vi "Servo Camera.vi"() -> ()   [LabVIEW 2013]
doc: "<B>Servo Camera Example</B> will track a colored object by moving a gimbal mounted camera to keep the object centered in the image. It assumes the camera is mounted upright, and that the DS is connected. It is written to control two servos, but will work fine with one. To tune the colors, you may find it easiest to set the Operation control to Camera Display. This way the servos will not update and you can experiment with the colors to get a good mask.\nOnce the color thresholds are set appropriately for the object you are tracking, switch Operation to GimbalTrack."
uses:
  <vilib>/addons/control/pid/NI_PID_pid.lvlib
  <vilib>/addons/control/pid/pid.llb/PID Control Input Filter (DBL).vi
  <vilib>/Rock Robotics/WPI/Camera/WPI_CameraFrameRate.ctl
  <vilib>/Rock Robotics/WPI/Camera/WPI_CameraImageSize.ctl
  Control States.ctl
  <vilib>/Rock Robotics/SystemInterfaces/DIO/FPGA_DIOPWMChannel.ctl
  2014 Target Detection/TargetType.ctl
panel:
  out "x = y?":cluster{bool, bool, bool, bool}
  in  "Color Components":T1={"Hue"={112.66304016113281, 144.6630401611328}, "Sat"={138.0, 255.0}, "Val"={139.0, 198.0}} {"Val" scale=0.0..255.0; "Sat" scale=0.0..255.0; "Hue" scale=0.0..255.0 scale format="%#_3g"}
  in  "Std Devs":cluster{"Hue":dbl, "Sat":dbl, "Val":dbl}={"Hue"=4.0, "Sat"=6.0, "Val"=4.0}
  out "Target Info":T3(array[cluster])
  in  "Score Cutoff":dbl(slide)=54.248366013071895 scale=0.0..100.0
  in  "Area Size Limit %":dbl=0.06 format="%#_13g"
  out "Image":T4(plugin-control)
  in  "stop":bool
  in  "Operation":enum32{"Camera Display", "Gimbal Track"}(radio)
  out "Servo Tracking State":T6
  in  "Servo Positions":cluster{"X":dbl, "Y":dbl}={"X"=85.52840986947938, "Y"=85.0} {"Y" scale=0.0..170.0; "X" scale=0.0..170.0}
  in  "Y Channel":T7=enum."PWM 5"
  in  "Loop Sleep":u32=20
  in  "Loop Sleep":u32=80
  in  "X Channel":T7=enum."PWM 4"
  in  "Image Decimation":cluster{"X":dbl, "Y":dbl}={"X"=5.0, "Y"=4.0}
  in  "Color Ranges":T8={"Hue"={"Min"=55, "Max"=93}, "Sat"={"Min"=41, "Max"=255}, "Luma"={"Min"=64, "Max"=255}}
  in  "Smooth":bool=TRUE
  out "Mask after threshold":T4(plugin-control)
  in  "Display Mask":bool=TRUE
  out "Camera Image":T4(plugin-control)
  # "This example will track a colored object by moving a gimbal mounted camera to keep the object centered in the image. It assumes the camera is mounted upright, and that the DS is connected. It is written to control two servos, but will work fine with one. To tune the colors, you may find it easiest to set the Operation control to Camera Display. This way the servos will not update and you can experiment with the colors to get a good mask.\nOnce the color thresholds are set appropriately for the object you are tracking, switch Operation to GimbalTrack."
  # "Servo Settings"
  # "Camera Settings"
  # "Hues are ~ 70, 150, and 250\nfor Green, Blue, and Red."
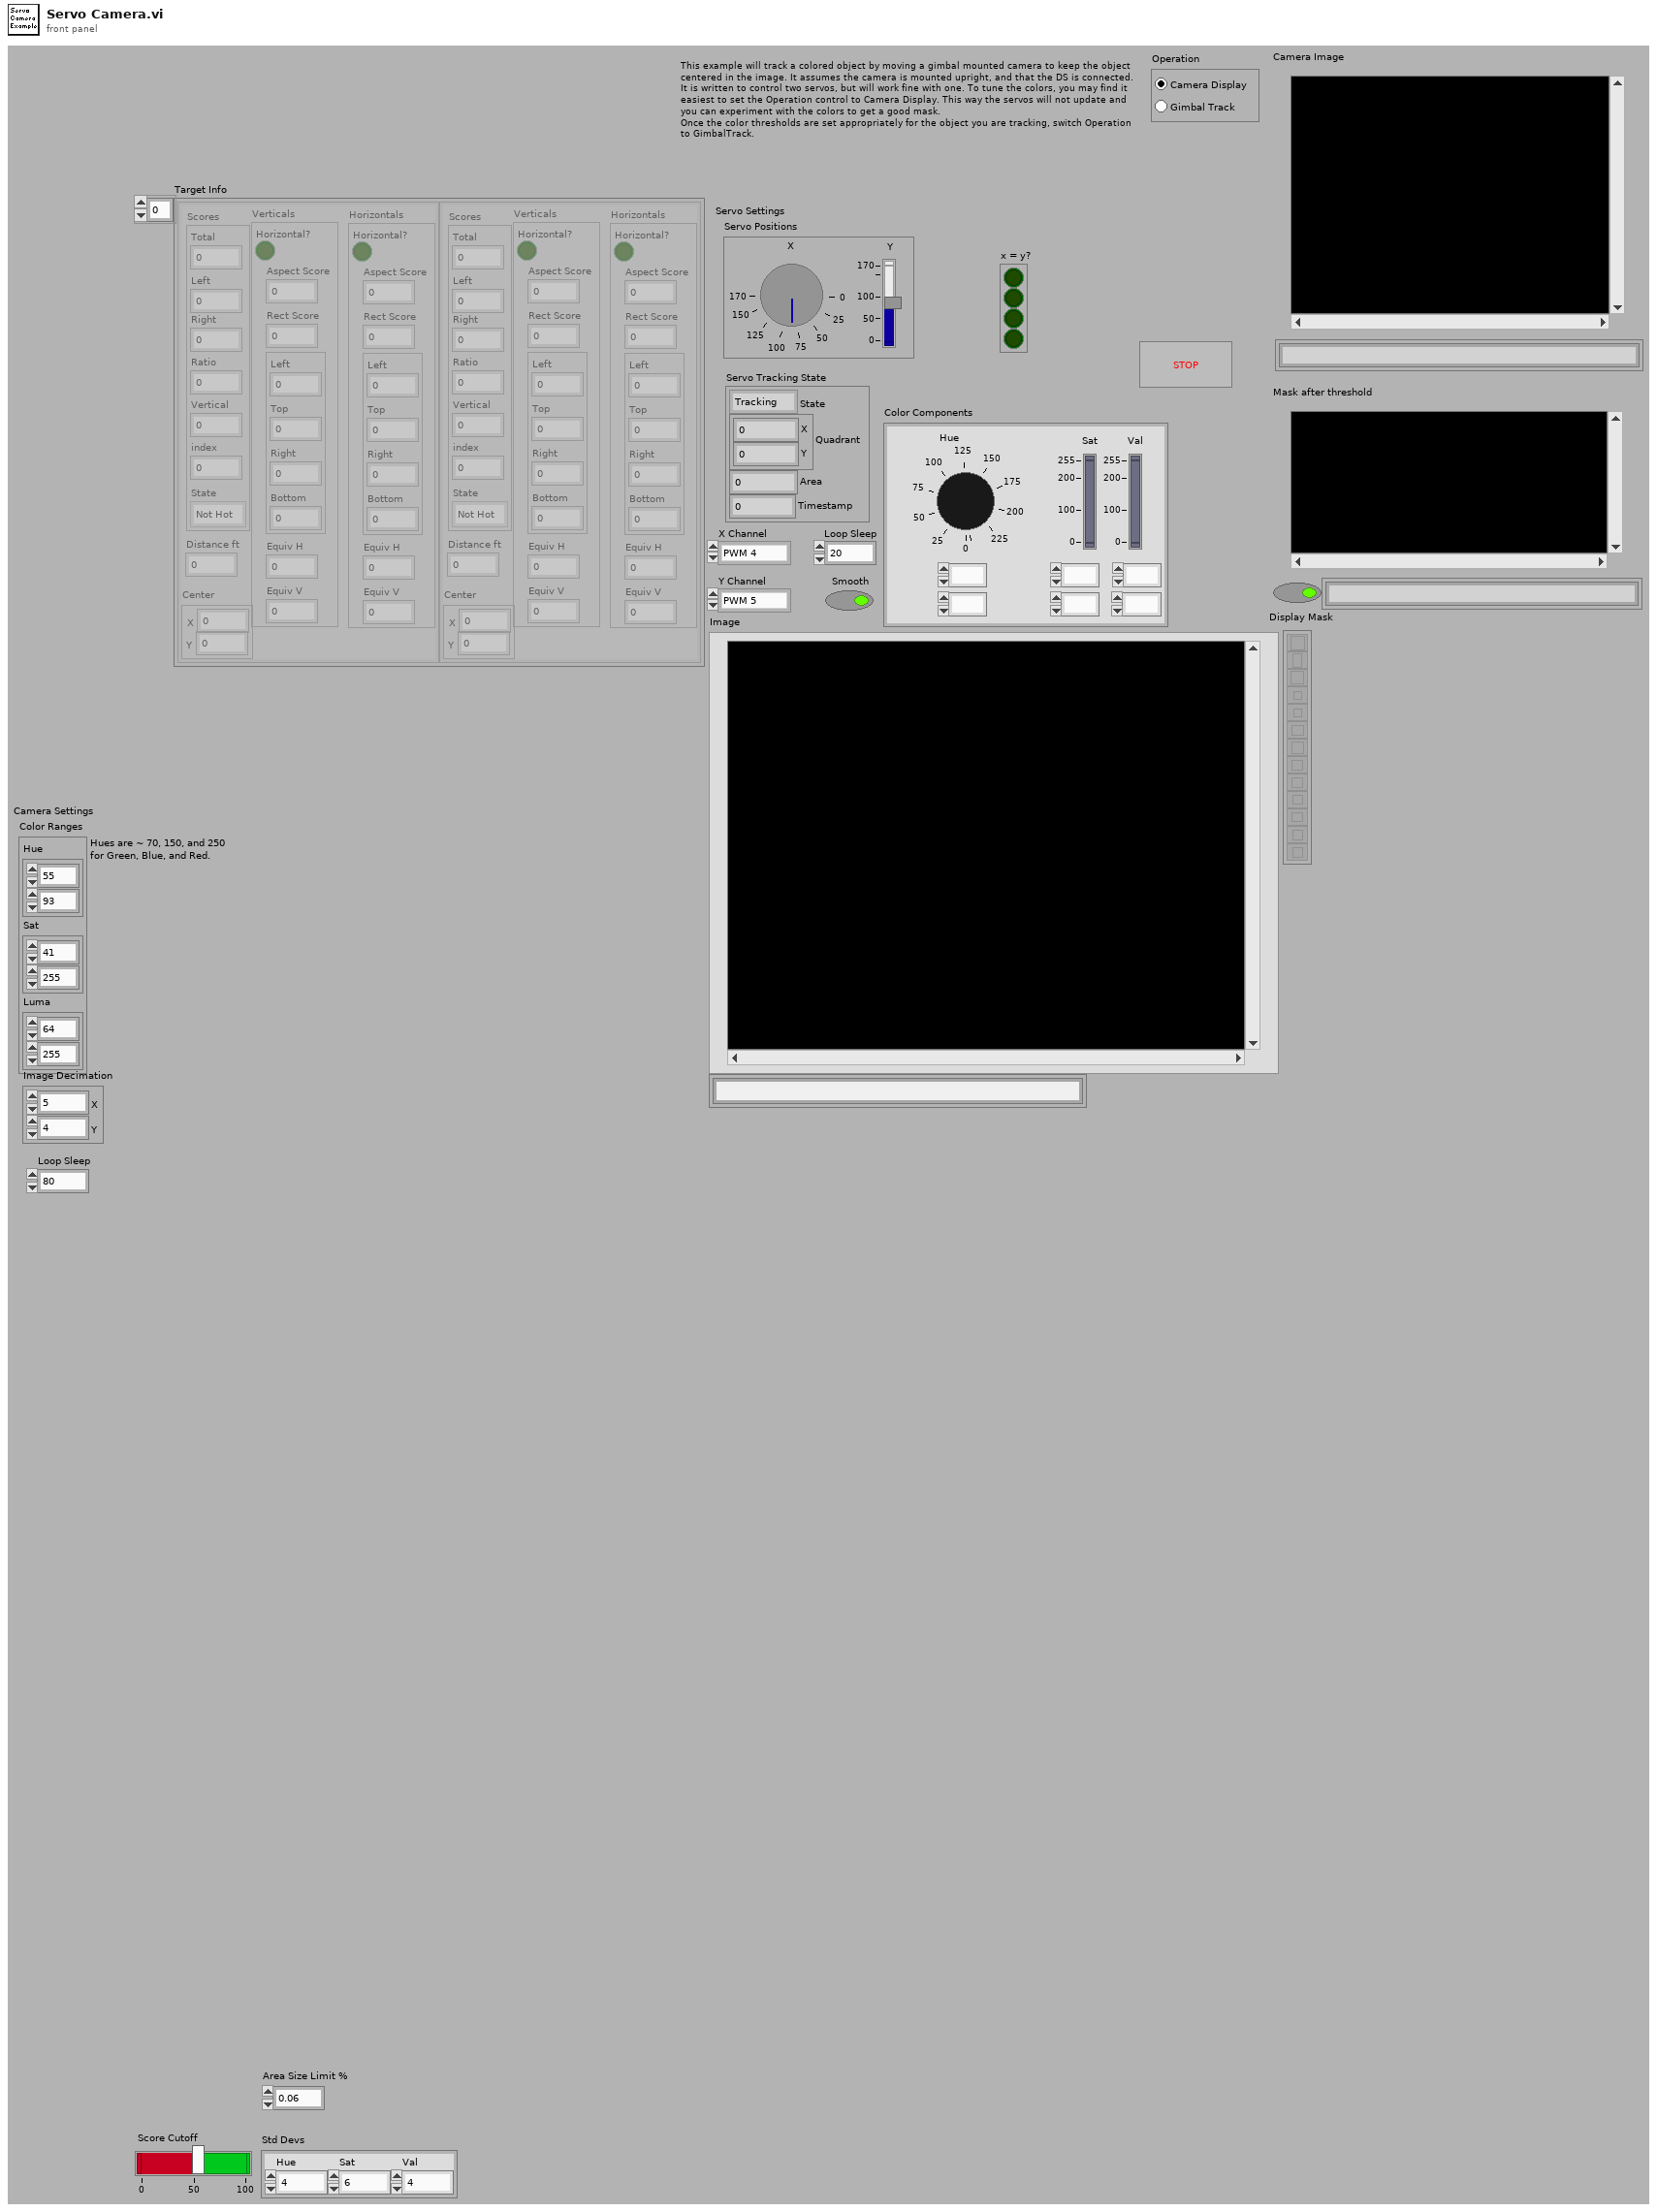
[diagram p1: front panel]
types:
  T1 = cluster{"Hue":cluster{dbl, dbl}, "Sat":cluster{dbl, dbl}, "Val":cluster{dbl, dbl}}
  T2 = typedef "TargetType.ctl" = enum16{"Not Hot", "Hot"}
  T3 = cluster{"Scores":cluster{"Total":dbl, "Left":dbl, "Right":dbl, "Ratio":dbl, "Vertical":dbl, "index":i32, "State":T2}, "Verticals":cluster{"Horizontal?":bool, "Aspect Score":dbl, "Rect Score":dbl, cluster{"Left":dbl, "Top":dbl, "Right":dbl, "Bottom":dbl}, "Equiv H":dbl, "Equiv V":dbl}, "Horizontals":cluster{"Horizontal?":bool, "Aspect Score":dbl, "Rect Score":dbl, cluster{"Left":dbl, "Top":dbl, "Right":dbl, "Bottom":dbl}, "Equiv H":dbl, "Equiv V":dbl}, "Distance ft":dbl, "Center":cluster{"X":dbl, "Y":dbl}}[]
  T4 = typedef "IMAQ Image.ctl" = refnum<image>
  T5 = typedef "Control States.ctl" = enum16{"Tracking", "Lost Small", "Lost-Patience", "Search-Begin", "Searching", "Lost - Edge"}
  T6 = cluster{"State":T5, "Quadrant":cluster{"X":i32, "Y":i32}, "Area":i32, "Timestamp":u32}
  T7 = typedef "FPGA_DIOPWMChannel.ctl" = enum8{"PWM 1", "PWM 2", "PWM 3", "PWM 4", "PWM 5", "PWM 6", "PWM 7", "PWM 8", "PWM 9", "PWM 10", "Invalid"}
  T8 = cluster{"Hue":cluster{"Min":i32, "Max":i32}, "Sat":cluster{"Min":i32, "Max":i32}, "Luma":cluster{"Min":i32, "Max":i32}}
  T9 = typedef "WPI_CameraImageSize.ctl" = enum16{"640x480", "320x240", "160x120"}
  T10 = typedef "WPI_CameraFrameRate.ctl" = u32
  T11 = typedef "WPI_CameraDevRef.ctl" = cluster{"Camera Address":string, "CameraStatus":errorcluster, "Acquire Image Notifier":refnum<notifier>}
  T12 = typedef "WPI_ServoDeviceRef.ctl" = cluster{"DeviceStatus":errorcluster, "Digital Module":T13, "PWM Channel":T7, "DeadBand":T14}
  T13 = typedef "FPGA_TypedefDigitalModule.ctl" = enum16{"Digital Module 1", "Digital Module 2"}
  T14 = typedef "WPI_PWMDeadband.ctl" = cluster{"Name":string, "maxPositivePwm":i32, "minPositivePwm":i32, "centerPwm":i32, "maxNegativePwm":i32, "minNegativePwm":i32, "angularRange":u16}
  T15 = cluster{"Left":i32, "Top":i32, "Right":i32, "Bottom":i32}
  T16 = cluster{"Horizontal":bool, "Aspect Score":dbl, "Rect Score":dbl, cluster{"Left":dbl, "Top":dbl, "Right":dbl, "Bottom":dbl}, "Equiv H":dbl, "Equiv V":dbl}[]
  T17 = cluster{cluster{dbl, dbl}, cluster{dbl, dbl}, cluster{dbl, dbl}}
  T18 = cluster{"Scores":cluster{"Total":dbl, "Left":dbl, "Right":dbl, "Ratio":dbl, "Vertical":dbl, "index":i32, "State":T2}, "Verticals":cluster{"Horizontal?":bool, "Aspect Score":dbl, "Rect Score":dbl, cluster{"Left":dbl, "Top":dbl, "Right":dbl, "Bottom":dbl}, "Equiv H":dbl, "Equiv V":dbl}, "Horizontals":cluster{"Horizontal?":bool, "Aspect Score":dbl, "Rect Score":dbl, cluster{"Left":dbl, "Top":dbl, "Right":dbl, "Bottom":dbl}, "Equiv H":dbl, "Equiv V":dbl}, "Validated":bool}[]
  T19 = cluster{"Distance (ft)":dbl, "Target Center (-1 to 1)":cluster{"X":dbl, "Y":dbl}, "Left":bool, "State":T2}[]
  T20 = cluster{"Scores":cluster{"Total":dbl, "Left":dbl, "Right":dbl, "Ratio":dbl, "Vertical":dbl, "index":i32, "State":T2}, "Verticals":cluster{"Horizontal?":bool, "Aspect Score":dbl, "Rect Score":dbl, cluster{"Left":dbl, "Top":dbl, "Right":dbl, "Bottom":dbl}, "Equiv H":dbl, "Equiv V":dbl}, "Horizontals":cluster{"Horizontal?":bool, "Aspect Score":dbl, "Rect Score":dbl, cluster{"Left":dbl, "Top":dbl, "Right":dbl, "Bottom":dbl}, "Equiv H":dbl, "Equiv V":dbl}, "Distance (ft)":dbl, "Target Center (-1 to 1)":cluster{"X":dbl, "Y":dbl}}[]
  T21 = cluster{"Scores":cluster{"Total":dbl, "Left":dbl, "Right":dbl, "Ratio":dbl, "Vertical":dbl, "index":i32, "State":T2}, "Verticals":cluster{"Horizontal?":bool, "Aspect Score":dbl, "Rect Score":dbl, cluster{"Left":dbl, "Top":dbl, "Right":dbl, "Bottom":dbl}, "Equiv H":dbl, "Equiv V":dbl}, "Horizontals":cluster{"Horizontal?":bool, "Aspect Score":dbl, "Rect Score":dbl, cluster{"Left":dbl, "Top":dbl, "Right":dbl, "Bottom":dbl}, "Equiv H":dbl, "Equiv V":dbl}, "Distance (ft)":dbl, "Target Center (-1 to 1)":cluster{"X":dbl, "Y":dbl}}
  T22 = cluster{"Horizontal?":bool, "Aspect Score":dbl, "Rect Score":dbl, cluster{"Left":dbl, "Top":dbl, "Right":dbl, "Bottom":dbl}, "Equiv H":dbl, "Equiv V":dbl}
  T23 = cluster{"Distance (ft)":dbl, "Target Center (-1 to 1)":cluster{"X":dbl, "Y":dbl}, "Left":bool, "State":T2}
  T24 = cluster{"Left":dbl, "Top":dbl, "Right":dbl, "Bottom":dbl}
  T25 = cluster{"State":T5, "Quadrant":cluster{"X":i32, "Y":i32}, "Area":i32, "millisecond timer value":u32}
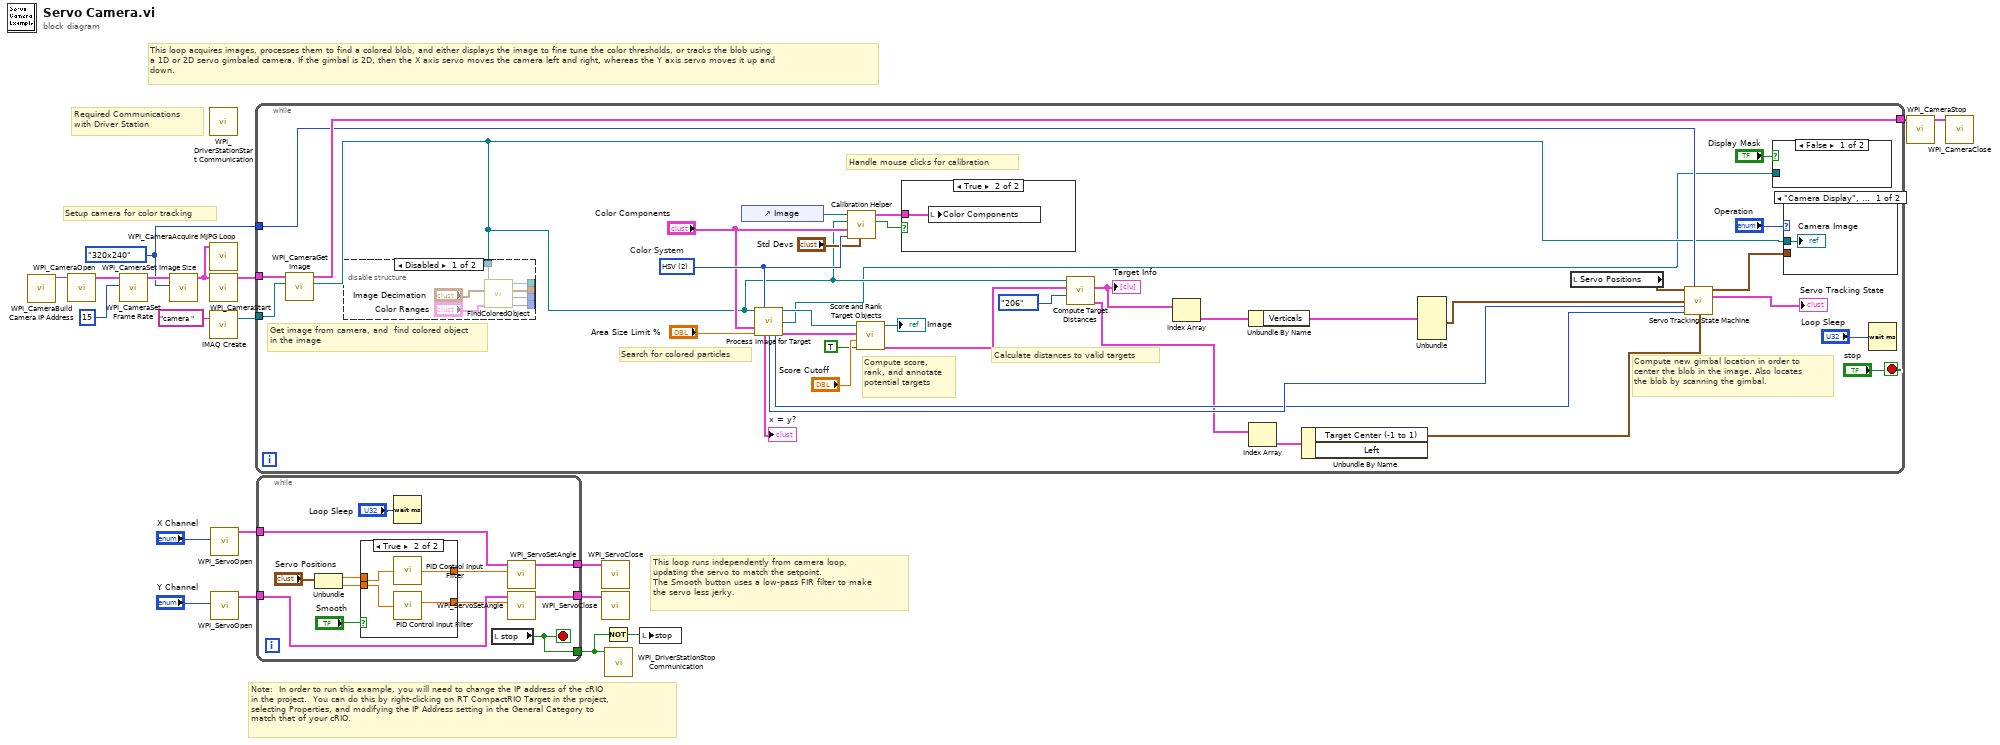
[diagram p0: block diagram]
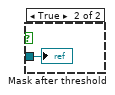
[diagram p4: hidden frame]
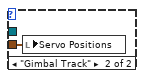
[diagram p5: hidden frame]
diagram:
  w7 = WPI_CameraImageSize."320x240" ("Image Size")
  # "Note:  In order to run this example, you will need to change the IP address of the cRIO\nin the project.  You can do this by right-clicking on RT CompactRIO Target in the project,\nselecting Properties, and modifying the IP Address setting in the General Category to \nmatch that of your cRIO."
  # "This loop acquires images, processes them to find a colored blob, and either displays the image to fine tune the color thresholds, or tracks the blob using\na 1D or 2D servo gimbaled camera. If the gimbal is 2D, then the X axis servo moves the camera left and right, whereas the Y axis servo moves it up and\ndown."
  # "This loop runs independently from camera loop,\nupdating the servo to match the setpoint.\nThe Smooth button uses a low-pass FIR filter to make\nthe servo less jerky."
  # "Setup camera for color tracking"
  # "Required Communications\nwith Driver Station"
  n1 = call <vilib>:"WPI_CameraBuild Camera IP Address.vi"() -> ("Camera Address"=w4:string)  [unwired: 11 in]
  n2 = call <vilib>:"WPI_CameraOpen.vi"("Camera Address"=w4) -> ("CameraDevRef"=w8:T11)  [unwired: 1 in, 9 out]
  n3 = call <vilib>:"WPI_CameraSet Frame Rate.vi"("Frame Rate (fps)"=T10 15, "CameraDevRef"=w8) -> ("CameraDevRef Out"=w9:T11)  [unwired: 1 in, 8 out]
  n4 = call <vilib>:"WPI_CameraSet Image Size.vi"("Image Size"=w7, "CameraDevRef"=w9) -> ("CameraDevRef Out"=w3:T11)  [unwired: 1 in, 8 out]
  n5 = call <vilib>:"WPI_DriverStationStart Communication.vi"() -> ()  [unwired: 1 in, 11 out]
  n6 = call <vilib>:"WPI_CameraAcquire MJPG Loop.vi"("CameraDevRef"=w3) -> ()  [unwired: 11 in]
  n7 = call <vilib>:"WPI_CameraStart.vi"("CameraDevRef"=w3) -> ("CameraDevRef Out"=w12:T11)  [unwired: 1 in, 9 out]
  n8 = call "IMAQ Create"("Image Name"="camera ") -> ("New Image"=w13:T4)  [unwired: 3 in, 2 out]
  n9 = call <vilib>:"WPI_ServoOpen.vi"("PWM Channel"="X Channel") -> ("ServoDeviceRef"=w17:T12)  [unwired: 3 in, 7 out]
  n10 = call <vilib>:"WPI_ServoOpen.vi"("PWM Channel"="Y Channel") -> ("ServoDeviceRef"=w16:T12)  [unwired: 3 in, 7 out]
  n11 = while {
    tunnel: w12 -> [w52]
    tunnel: [w51] -> w11
    tunnel: w13 -> [w55]
    tunnel: w7 -> [w46]
    stop <- "stop" stop-if-true
    w37 = u16 2 items=["RGB", "HSL", "HSV", "HSI"]  # Color System
    # "Calculate distances to valid targets"
    # "Search for colored particles"
    # "Handle mouse clicks for calibration"
    # "Compute score,\nrank, and annotate\npotential targets"
    # "Compute new gimbal location in order to\ncenter the blob in the image. Also locates\nthe blob by scanning the gimbal."
    # "Get image from camera, and  find colored object in the image"
    n12 = call <vilib>:"WPI_CameraGet Image.vi"("Image"=w55, "CameraDevRef"=w52) -> ("Image Out"=w31:T4, "CameraDevRef Out"=w51:T11)  [unwired: 1 in, 7 out]
    n13 = disable-structure shown="Disabled" {
      disable-tunnel: [w64 _] -> _
      disable-tunnel: [w63 _] -> _
      disable-tunnel: [w62 _] -> _
      disable-tunnel: [w59 _] -> _
      disable-tunnel: w31 -> [w58 _]
      frame Disabled {
        n14 = call "FindColoredObject.vi"("Color Range"="Color Ranges", "Decimate by"="Image Decimation", "Color Image In"=w58) -> ("Area"=w62:i32, "Particles"=w63:i32, "Rectangle"=w64:T15, "Mask Image"=w59:T4)  [unwired: 3 out]
      }
      frame Enabled {
      }
    }
    n15 = control-ref of="Image"() -> (w38:refnum<vi>)
    n16 = call "Process Image for Target.vi"("Src Image"=w31, "Color Mode"=w37, "Color Components"="Color Components", "Area Cutoff %"="Area Size Limit %") -> ("Src Image Out"=w44:T4, "Threshold"=w30:T4, "x = y?"=→"x = y?":cluster{bool, bool, bool, bool}, "Particles gimbal"=w25:i32, "area"=w24:i32, "Particles"=w41:T16)  [unwired: 6 in]
    n17 = call "Calibration Helper.vi"("Std Devs"="Std Devs", "Color Mode"=w37, "Color Components"="Color Components", "Image"=w31, "Image Ctl Refnum"=w38) -> ("Changed"=w33:bool, "output color"=w35:T17)  [unwired: 5 in]
    n18 = call "Score and Rank Target Objects.vi"("Annotate"=TRUE, "Score Limit"="Score Cutoff", "Particles"=w41, "Image in"=w44) -> ("Target Info"=w40:T18, "Annotated Image"=→"Image":T4)  [unwired: 6 in]
    n19 = case shown="True" w33 {
      tunnel: w35 -> [_ w57]
      frame False {
      }
      frame True {
        n20 = local write "Color Components"(w57) -> ()
      }
    }
    n21 = call "Compute Target Distances.vi"("Camera Type"=enum16{"206", "1011", "1013"}."206", "Target Info"=w40, "Image in"=w31) -> ("Distances"=w22:T19, "Target Info"=w29:T20)  [unwired: 6 in, 1 out]
    "Target Info" <- w29
    n22 = Index Array(array=w29) -> (element=w28:T21)  [unwired: 1 in]
    n23 = Unbundle By Name(w28) -> ("Verticals"=w27:T22)
    n24 = Index Array(array=w22) -> (element=w21:T23)  [unwired: 1 in]
    n25 = Unbundle By Name(w21) -> ("Target Center (-1 to 1)"=w20:cluster{"X":dbl, "Y":dbl})  [unwired: 1 out]
    n26 = Unbundle(w27) -> (w26:T24)  [unwired: 5 out]
    n27 = local read "Servo Positions"() -> (w50:cluster{"X":dbl, "Y":dbl})
    n28 = call "Servo Tracking State Machine.vi"("Servo Positions In"=w50, "Image Size"=w46, "Rectangle"=w26, "Particles"=w25, "Area"=w24, "Center"=w20) -> ("Servo Positions"=w54:cluster{"X":dbl, "Y":dbl}, "Tracking State Info"=→"Servo Tracking State":T25)  [unwired: 1 in, 7 out]
    n29 = case shown="False" "Display Mask" {
      tunnel: w30 -> [_ w65]
      frame False {
      }
      frame True {
        "Mask after threshold" <- w65
      }
    }
    n30 = case shown="\"Camera Display\", Default" "Operation" {
      tunnel: w54 -> [_ w67]
      tunnel: w31 -> [w66 _]
      frame "Camera Display", Default {
        "Camera Image" <- w66
      }
      frame "Gimbal Track" {
        n31 = local write "Servo Positions"(w67) -> ()
      }
    }
    n32 = Wait (ms)(milliseconds to wait="Loop Sleep") -> ()  [unwired: 1 out]
  }
  n33 = while {
    tunnel: w17 -> [w77]
    tunnel: [w79] -> w6
    tunnel: w16 -> [w76]
    tunnel: [w75] -> w5
    tunnel: [w68] -> w2
    stop <- w68 stop-if-true
    n34 = Unbundle("Servo Positions") -> ("X"=w73:dbl, "Y"=w71:dbl)
    n35 = case shown="True" "Smooth" {
      tunnel: w73 -> [w81 w85]
      tunnel: [w81 w84] -> w72
      tunnel: w71 -> [w80 w83]
      tunnel: [w80 w82] -> w70
      frame False {
      }
      frame True {
        n36 = call-poly <vilib>:"PID Control Input Filter.vi"("input"=w85) -> ("output"=w84:dbl)  [unwired: 1 in, 3 out]
        n37 = call-poly <vilib>:"PID Control Input Filter.vi"("input"=w83) -> ("output"=w82:dbl)  [unwired: 1 in, 3 out]
      }
    }
    n38 = Wait (ms)(milliseconds to wait="Loop Sleep") -> ()  [unwired: 1 out]
    n39 = local read "stop"() -> (w68:bool)
    n40 = call <vilib>:"WPI_ServoSetAngle.vi"("Angle"=w72, "ServoDeviceRef"=w77) -> ("ServoDeviceRef"=w79:T12)  [unwired: 1 in, 8 out]
    n41 = call <vilib>:"WPI_ServoSetAngle.vi"("Angle"=w70, "ServoDeviceRef"=w76) -> ("ServoDeviceRef"=w75:T12)  [unwired: 1 in, 8 out]
  }
  n42 = call <vilib>:"WPI_ServoClose.vi"("MotorControlDevRef"=w6) -> ()  [unwired: 1 in, 10 out]
  n43 = call <vilib>:"WPI_ServoClose.vi"("MotorControlDevRef"=w5) -> ()  [unwired: 1 in, 10 out]
  n44 = Not(x=w2) -> (.not. x?=w1:bool)
  n45 = call <vilib>:"WPI_DriverStationStop Communication.vi"("StopCommunication"=w2) -> ()  [unwired: 1 in, 10 out]
  n46 = local write "stop"(w1) -> ()
  n47 = call <vilib>:"WPI_CameraStop.vi"("CameraDevRef"=w11) -> ("CameraDevRef Out"=w15:T11)  [unwired: 1 in, 9 out]
  n48 = call <vilib>:"WPI_CameraClose.vi"("CameraDevRef"=w15) -> ()  [unwired: 1 in, 10 out]
